vi "To Variant.vi"(8 "error in (no error)":errorcluster, 11 "Abs_Value in":refnum<class "Abs_Value.lvclass">) -> (0 "error out":errorcluster, 2 "Variant":variant, 3 "Abs_Value out":refnum<class "Abs_Value.lvclass">)   [LabVIEW 2021, in "Abs_Value.lvclass"]
uses:
  Abs_Value.lvclass
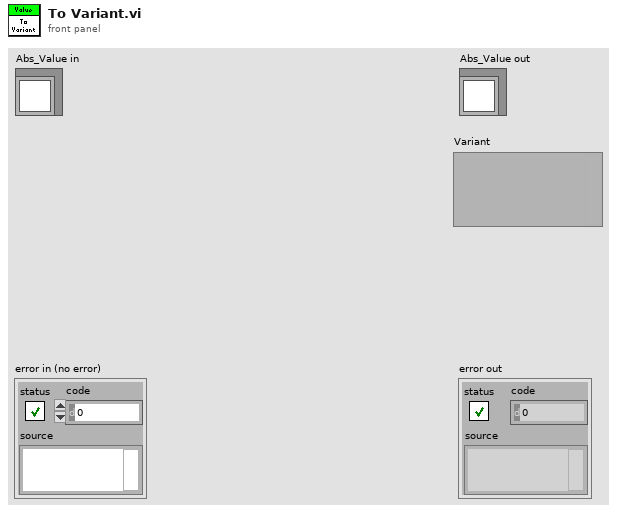
[diagram p1: front panel]
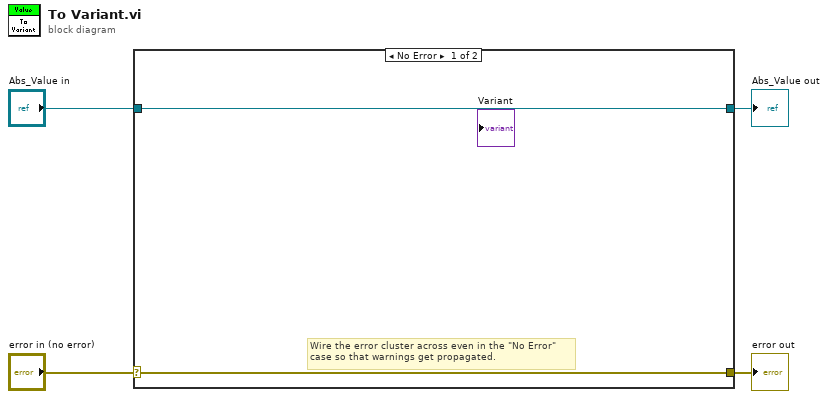
[diagram p0: block diagram]
diagram:
  n1 = case shown="No Error" "error in (no error)" {
    selector: "error in (no error)" -> [w5 w8]
    tunnel: [w5 w8] -> w3
    tunnel: [w6 w7] -> w1
    tunnel: "Abs_Value in" -> [w6 w7]
    frame No Error {
      # "Wire the error cluster across even in the \"No Error\"\ncase so that warnings get propagated."
    }
    frame Error {
    }
  }
  "error out" <- w3
  "Abs_Value out" <- w1
